vi "Initialize Subpanels.vi"(8 "error in (no error)":errorcluster, 11 "UI Controller in":refnum<class "UI Controller.lvclass">) -> (0 "error out":errorcluster, 3 "UI Controller out":refnum<class "UI Controller.lvclass">)   [LabVIEW 2015, in "UI Controller.lvlib" / "UI Controller.lvclass"]
uses:
  UI Controller.lvclass
  <vilib>/Utility/miscctls.llb/LVPositionTypeDef.ctl
  <vilib>/ActorFrameworkMVC/View Controller/View Controller/View Controller.lvclass
panel:
  # "NOTICE -- YOU MUST LEAVE THIS NOTICE IN PLACE.\n\nCopyright (c) 2015, LIANG LIU Shawn.Liu.cn@gmail.com\nAll rights reserved.\n\nRedistribution and use in source and binary forms, with or without modification, are permitted provided that the following conditions are met:\n-Redistributions of source code must retain the above copyright notice, this list of conditions and the following disclaimer.\n-Redistributions in binary form must reproduce the above copyright notice, this list of conditions and the following disclaimer in the documentation and/or other materials provided with the distribution.\n-Neither the name of the eLp nor the names of its contributors may be used to endorse or promote products derived from this software without specific prior written permission.\n\nTHIS SOFTWARE IS PROVIDED BY THE COPYRIGHT HOLDERS AND CONTRIBUTORS \"AS IS\" AND ANY EXPRESS OR IMPLIED WARRANTIES, INCLUDING, BUT NOT LIMITED TO, THE IMPLIED WARRANTIES OF MERCHANTABILITY AND FITNESS FOR A PARTICULAR PURPOSE ARE DISCLAIMED. IN NO EVENT SHALL THE COPYRIGHT HOLDER OR CONTRIBUTORS BE LIABLE FOR ANY DIRECT, INDIRECT, INCIDENTAL, SPECIAL, EXEMPLARY, OR CONSEQUENTIAL DAMAGES (INCLUDING, BUT NOT LIMITED TO, PROCUREMENT OF SUBSTITUTE GOODS OR SERVICES; LOSS OF USE, DATA, OR PROFITS; OR BUSINESS INTERRUPTION) HOWEVER CAUSED AND ON ANY THEORY OF LIABILITY, WHETHER IN CONTRACT, STRICT LIABILITY, OR TORT (INCLUDING NEGLIGENCE OR OTHERWISE) ARISING IN ANY WAY OUT OF THE USE OF THIS SOFTWARE, EVEN IF ADVISED OF THE POSSIBILITY OF SUCH DAMAGE."
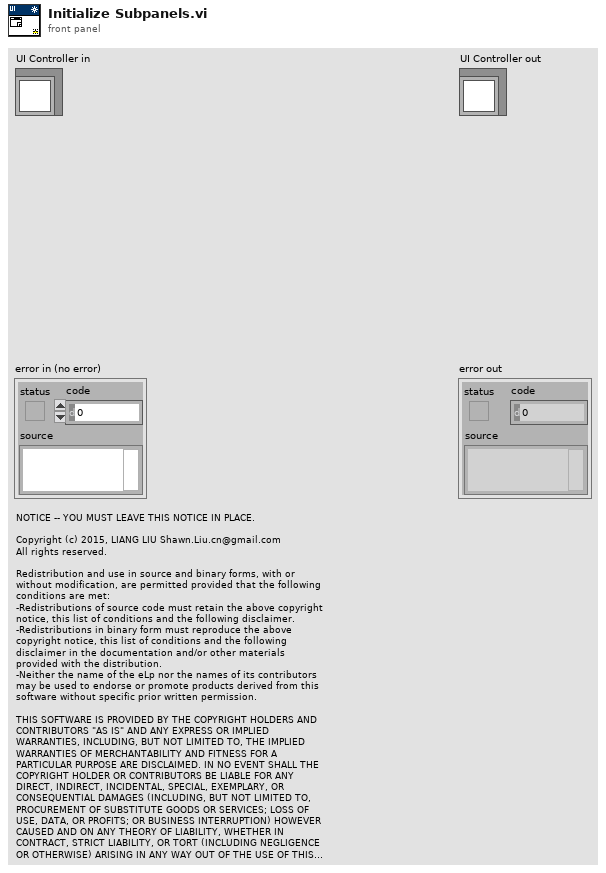
[diagram p1: front panel]
types:
  T1 = typedef "LVPositionTypeDef.ctl" = cluster{"Left":i32, "Top":i32}
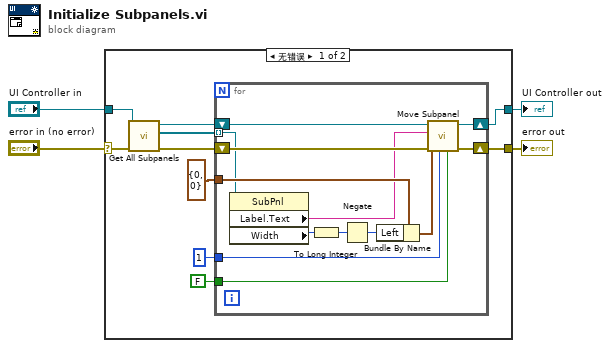
[diagram p0: block diagram]
diagram:
  n1 = case shown="无错误" "error in (no error)" {
    selector: "error in (no error)" -> [w13 w29]
    tunnel: "UI Controller in" -> [w5 w28]
    tunnel: [w8 w29] -> w2
    tunnel: [w7 w28] -> w1
    frame No Error {
      n2 = call <vilib>:"Get All Subpanels.vi"("error in (no error)"=w13, "View Controller in"=w5) -> ("error out"=w10:errorcluster, "Subpanels"=w6:refnum<vi>[], "View Controller out"=w9:refnum<class "UI Controller.lvclass">)  [unwired: 7 in]
      n3 = for {
        tunnel: T1 {"Left"=0, "Top"=0} ("Position") -> [w26]
        tunnel: 1 ("Loop Number (16)") -> [w25]
        tunnel: FALSE ("Visible (True)") -> [w24]
        shift-right: [w21] -> w8
        shift-left: w10 -> [w23]
        shift-right: [w20] -> w7
        shift-left: w9 -> [w22]
        tunnel: w6 -> [w19] mode=indexing
        n4 = property class="SubPnl"(reference=w19) -> ("Label.Text"=w15:string, "Width"=w17:u32)  [unwired: 1 in, 2 out]
        n5 = To Long Integer(number=w17) -> (32bit integer=w16:i32)
        n6 = Negate(x=w16) -> (-x=w18:i32)
        n7 = Bundle By Name(cluster=w26, "Left"=w18) -> (w27:T1)
        n8 = call-dynamic "Move Subpanel.vi"("Visible (True)"=w24, "Loop Number (16)"=w25, "error in (no error)"=w23, "Position"=w27, "Subpanel Name"=w15, "UI Controller in"=w22) -> ("error out"=w21:errorcluster, "UI Controller out"=w20:refnum<class "UI Controller.lvclass">)  [unwired: 4 in]
      }
    }
    frame Error {
    }
  }
  "error out" <- w2
  "UI Controller out" <- w1
